vi "Test_AddGetTopic_RetrievalOK.vi"(8 "error in (no error)":errorcluster, 11 "TestCase in":refnum<class "TestTopicLookupTable.lvclass">) -> (0 "error out":errorcluster, 3 "TestCase out":refnum<class "TestTopicLookupTable.lvclass">)   [LabVIEW 2020, in "TestTopicLookupTable.lvclass"]
uses:
  TestTopicLookupTable.lvclass
  TestTopicLookupTable.lvclass/TestTopicLookupTable.ctl
  Source/Mediator/TopicLookupTable/TopicLookupTable.lvclass
  Source/Mediator/Topic/Topic.lvclass
  <vilib>/ActorFramework/Message Queue/Message Queue.lvclass
  <vilib>/ActorFramework/Message Enqueuer/Message Enqueuer.lvclass
  modules/composed-event-logger/Source/Composed Log/LoggerReference/LoggerReference.lvclass
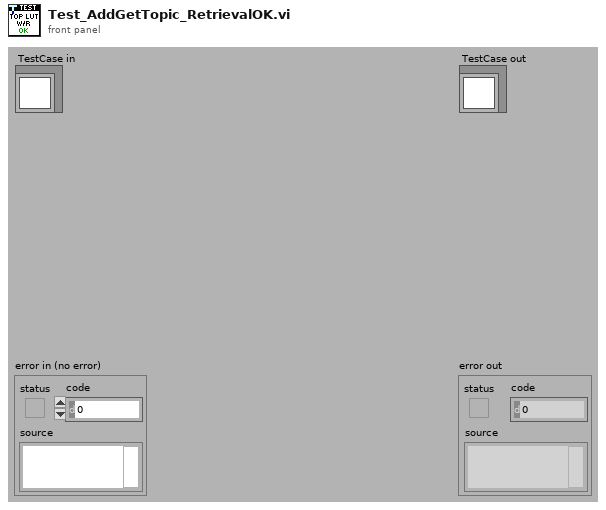
[diagram p1: front panel]
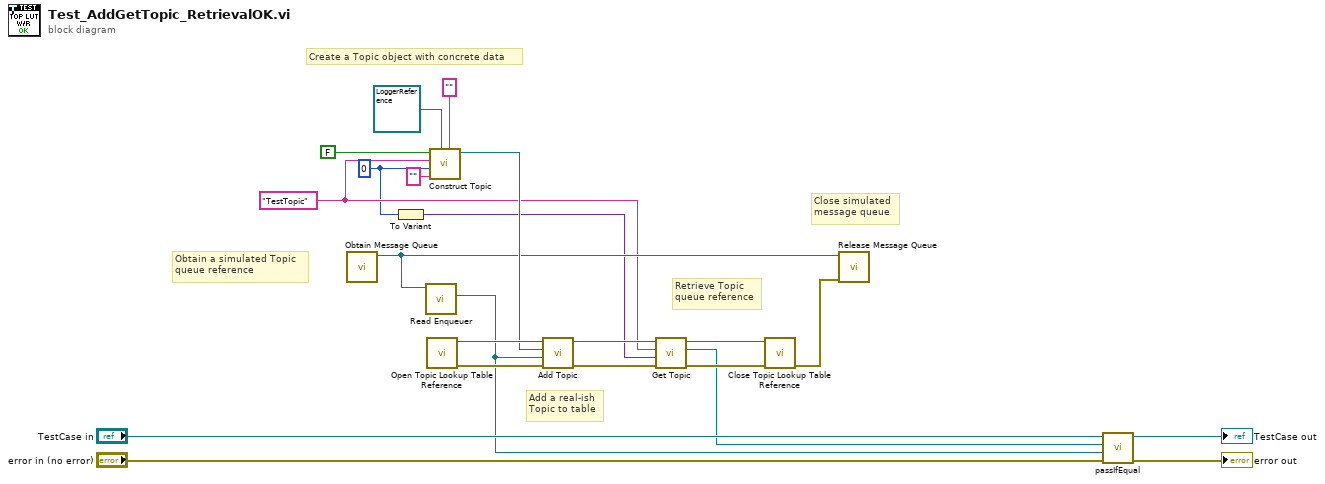
[diagram p0: block diagram]
diagram:
  w7 = 0
  w8 = "TestTopic" ("Name")
  # "Create a Topic object with concrete data"
  # "Add a real-ish\nTopic to table"
  # "Close simulated\nmessage queue"
  # "Retrieve Topic\nqueue reference"
  # "Obtain a simulated Topic\nqueue reference"
  n1 = call <vilib>:"Obtain Message Queue.vi"() -> ("Message Queue"=w9:refnum<class "Message Queue.lvclass">)  [unwired: 10 in, 1 out]
  n2 = To Variant(anything=w7) -> (Variant=w6:variant)
  n3 = call <vilib>:"Read Enqueuer.vi"("Message Queue"=w9) -> ("Message Enqueuer"=w11:refnum<class "Message Enqueuer.lvclass">)  [unwired: 10 in]
  n4 = call "Open Topic Lookup Table Reference.vi"() -> ("error out"=w17:errorcluster, "TopicLookupTable Reference"=w18:refnum<data-value>)  [unwired: 10 in]
  n5 = call "Construct Topic.vi"("Framework Instance Alias"="", "Event Log Instance"=refnum<class "LoggerReference.lvclass"> refnum, "Lock Owner ID (\"\" = NOT Locked)"="" ("Lock Owner ID (\"\" = NOT Locked)"), "New Topic Data"=w7, "Name"=w8, "Use Type Input As Initial Value?"=FALSE) -> ("Topic out"=w12:refnum<class "Topic.lvclass">)  [unwired: 4 in, 1 out]
  n6 = call "Add Topic.vi"("error in (no error)"=w17, "Topic Enqueuer"=w11, "Topic Object"=w12, "TopicLookupTable"=w18) -> ("error out"=w15:errorcluster, "TopicLookupTable"=w16:refnum<data-value>)  [unwired: 5 in, 1 out]
  n7 = call "Get Topic.vi"("error in (no error)"=w15, "Topic Type"=w6, "Topic Name"=w8, "TopicLookupTable"=w16) -> ("error out"=w13:errorcluster, "Topic Enqueuer"=w5:refnum<class "Message Enqueuer.lvclass">, "TopicLookupTable"=w14:refnum<data-value>)  [unwired: 5 in]
  n8 = call "Close Topic Lookup Table Reference.vi"("error in (no error)"=w13, "TopicLookupTable"=w14) -> ("error out"=w10:errorcluster)  [unwired: 9 in]
  n9 = call <vilib>:"Release Message Queue.vi"("error in (no error)"=w10, "Message Queue"=w9) -> ()  [unwired: 8 in, 2 out]
  n10 = call-dynamic "passIfEqual.vi"("error in (no error)"="error in (no error)", "y"=w11, "x"=w5, "TestCase in"="TestCase in") -> ("error out"=→"error out":errorcluster, "TestCase out"=→"TestCase out":refnum<class "TestTopicLookupTable.lvclass">)  [unwired: 6 in]
